vi "Open Screenpop.vi"(5 "Screenpop URL Prefix":string, 7 "SR# Cloumn Header":string, 9 "Coordinates":T1, 11 "Table Reference":refnum<vi>) -> ()   [LabVIEW 2017, in "Client.lvlib"]
uses:
  Client.lvlib
  <vilib>/Utility/miscctls.llb/LVPoint32TypeDef.ctl
  <vilib>/Platform/browser.llb/Open URL in Default Browser (string).vi
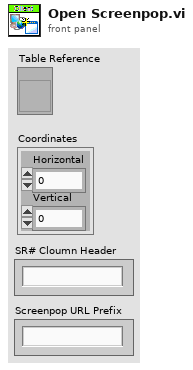
[diagram p1: front panel]
types:
  T1 = typedef "LVPoint32TypeDef.ctl" = cluster{"Horizontal":i32, "Vertical":i32}
  T2 = typedef "LVRowAndColumnTypeDef.ctl" = cluster{"Row":i32, "Column":i32}
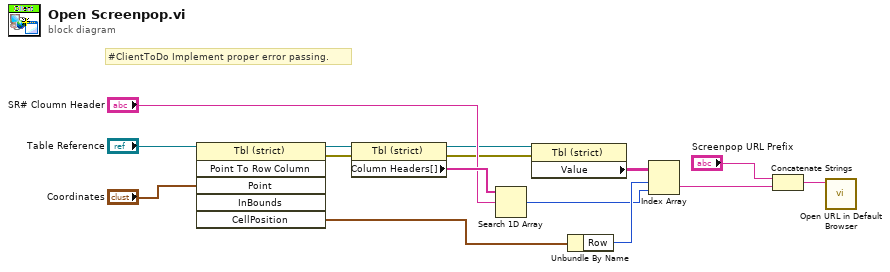
[diagram p0: block diagram]
diagram:
  # "#ClientToDo Implement proper error passing."
  n1 = invoke class="Tbl (strict)" method="Point To Row Column"(reference="Table Reference", "Point"="Coordinates") -> (reference out=w12:refnum<vi>, error out=w8:errorcluster, "CellPosition"=w15:T2)  [unwired: 4 in, 3 out]
  n2 = property class="Tbl (strict)"(reference=w12, error in=w8) -> (reference out=w9:refnum<vi>, error out=w7:errorcluster, "Column Headers[]"=w11:string[])
  n3 = Search 1D Array(1D array=w11, element="SR# Cloumn Header") -> (index of element=w4:i32)  [unwired: 1 in]
  n4 = property class="Tbl (strict)"(reference=w9, error in=w7) -> ("Value"=w6:string[][])  [unwired: 2 out]
  n5 = Unbundle By Name(w15) -> ("Row"=w5:i32)
  n6 = Index Array(array=w6, index (row)=w5, index (col)=w4) -> (element=w2:string)
  n7 = Concatenate Strings("Screenpop URL Prefix", w2) -> (w1:string)
  n8 = call-poly <vilib>:"Open URL in Default Browser.vi"("URL"=w1) -> ()  [unwired: 5 in, 2 out]
